vi "HGF_Timing.appendData2Variant.vi"(0 "initData":variant, 3 "defaultObject":refnum<class>, 5 "error in (no error)":errorcluster) -> (14 "dup initData":variant, 19 "error out":errorcluster)   [LabVIEW 2014, in "HGF_BaseClasses.lvlib" / "HGF_Timing.lvclass"]
doc: "Append initialize data to variant."
uses:
  HGF_Timing.lvclass
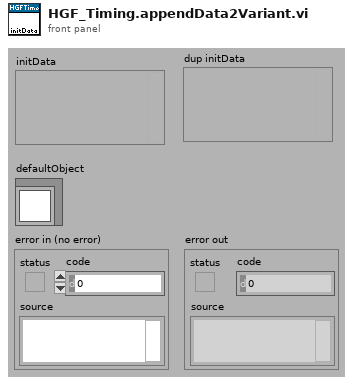
[diagram p1: front panel]
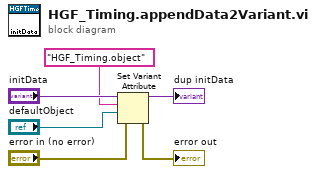
[diagram p0: block diagram]
diagram:
  n1 = Set Variant Attribute(Variant="initData", name="HGF_Timing.object", value="defaultObject", error in="error in (no error)") -> (Variant out=→"dup initData":variant, error out=→"error out":errorcluster)  [unwired: 1 out]
